vi "Get Measurement Auto Range Lower Limit.vi"(0 "VISA resource name":refnum<visa-resource-name>, 11 "error in (no error)":errorcluster) -> (4 "VISA resource name out":refnum<visa-resource-name>, 6 "Voltage AutoRange Lower Limit":dbl, 8 "Current AutoRange Lower Limit":dbl, 10 "Resistance AutoRange Lower Limit":dbl, 15 "error out":errorcluster)   [LabVIEW 2017, in "Keithley 2450.lvlib"]
doc: "Gets the measurement auto range lower limit for V, I and R on the instrument."
uses:
  Keithley 2450.lvlib
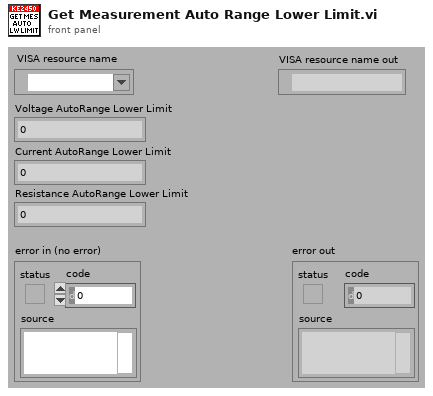
[diagram p1: front panel]
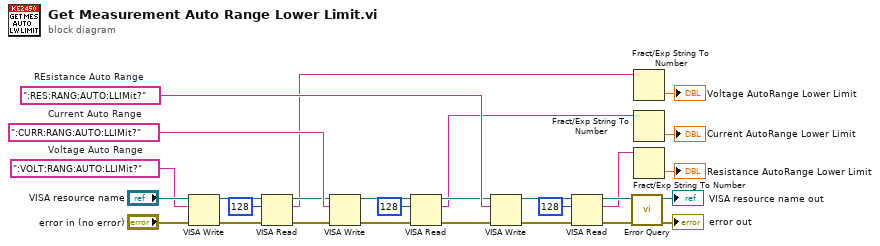
[diagram p0: block diagram]
diagram:
  w10 = ":RES:RANG:AUTO:LLIMit?"  # REsistance Auto Range
  w11 = ":CURR:RANG:AUTO:LLIMit?"  # Current Auto Range
  w12 = ":VOLT:RANG:AUTO:LLIMit?"  # Voltage Auto Range
  n1 = VISA Write(VISA resource name="VISA resource name", write buffer=w12, error in (no error)="error in (no error)") -> (VISA resource name out=w27:refnum<visa-resource-name>, error out=w28:errorcluster)  [unwired: 1 out]
  n2 = VISA Read(VISA resource name=w27, byte count=u32 128, error in (no error)=w28) -> (VISA resource name out=w8:refnum<visa-resource-name>, read buffer=w3:string, error out=w14:errorcluster)  [unwired: 1 out]
  n3 = VISA Write(VISA resource name=w8, write buffer=w11, error in (no error)=w14) -> (VISA resource name out=w20:refnum<visa-resource-name>, error out=w19:errorcluster)  [unwired: 1 out]
  n4 = VISA Read(VISA resource name=w20, byte count=u32 128, error in (no error)=w19) -> (VISA resource name out=w9:refnum<visa-resource-name>, read buffer=w2:string, error out=w15:errorcluster)  [unwired: 1 out]
  n5 = VISA Write(VISA resource name=w9, write buffer=w10, error in (no error)=w15) -> (VISA resource name out=w17:refnum<visa-resource-name>, error out=w18:errorcluster)  [unwired: 1 out]
  n6 = VISA Read(VISA resource name=w17, byte count=u32 128, error in (no error)=w18) -> (VISA resource name out=w7:refnum<visa-resource-name>, read buffer=w1:string, error out=w13:errorcluster)  [unwired: 1 out]
  n7 = call "Error Query.vi"("error in (no error)"=w13, "VISA resource name"=w7) -> ("error out"=→"error out":errorcluster, "VISA resource name out"=→"VISA resource name out":refnum<visa-resource-name>)  [unwired: 8 out]
  n8 = Fract/Exp String To Number(string=w3) -> (number=→"Voltage AutoRange Lower Limit":dbl)  [unwired: 3 in, 1 out]
  n9 = Fract/Exp String To Number(string=w2) -> (number=→"Current AutoRange Lower Limit":dbl)  [unwired: 3 in, 1 out]
  n10 = Fract/Exp String To Number(string=w1) -> (number=→"Resistance AutoRange Lower Limit":dbl)  [unwired: 3 in, 1 out]
